vi "FILE New.vi"(0 "New File Path":path, 1 "Prompt":string, 2 "Pattern":string, 3 "Default Name":string, 7 "Append Mode (Overwrite)":T2, 11 "Error In (no error)":errorcluster, 12 "Start Path":path, 13 "Warn on Overwrite (warn)":T1) -> (4 "Refnum":refnum<file>, 8 "File Path":path, 15 "Error Out":errorcluster)   [LabVIEW 2011]
doc: "This vi initializes the creation of a new file, the overwriting of an old file, or the append of new information to an old file depending on the mode enumerations specified.\n\nappend mode: controls the mode that the write operation will take if the file path already exhists. If append is selected then the text (or spreadsheed array) will be appended to the data after the last character in the file. If overwrite is selected then the file will be overwritten by the new data specified.\n\nwarning dialog mode : controls the action of the dialog to warn when a file is about to be overwritten. If 'don't warn' is selected then the file will be automatically overwritten. If the dialog appears and the user chooses not to overwrite then no file operation will take place and no errors will ocurr.\n\nnote: generally canceling out of all dialog boxes will not cause a file error to ocurr, only actual file errors will be flagged."
uses:
  Type Defs/FILE Append Mode Enum.ctl
  Type Defs/FILE Overwrite Warning Enum.ctl
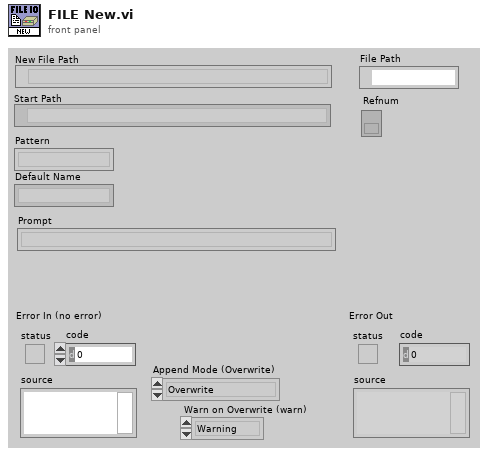
[diagram p1: front panel]
types:
  T1 = typedef "FILE Overwrite Warning Enum.ctl" = enum16{"Warning", "No Warning"}
  T2 = typedef "FILE Append Mode Enum.ctl" = enum16{"Overwrite", "Append"}
  T3 = enum16{"open", "replace", "create", "open or create", "replace or create", "replace or create with confirmation"}
  T4 = enum32{"existing file", "new file", "new or existing file", "existing dir", "new dir", "new or existing dir", "existing file (use LLBs)", "new file (use LLBs)", "new or existing file (use LLBs)", "new or existing file or directory (use LLBs)"}
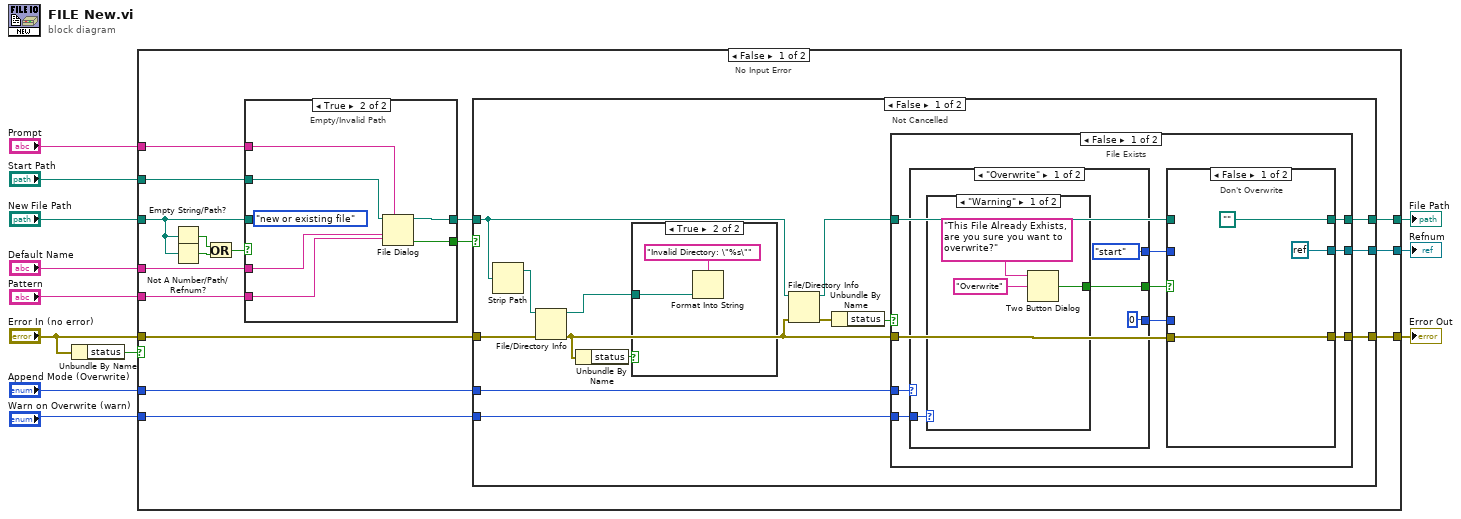
[diagram p0: block diagram]
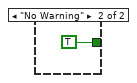
[diagram p3: hidden frame]
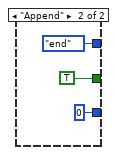
[diagram p4: hidden frame]
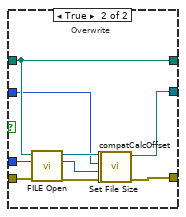
[diagram p5: hidden frame]
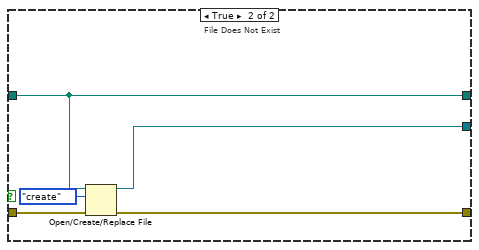
[diagram p6: hidden frame]
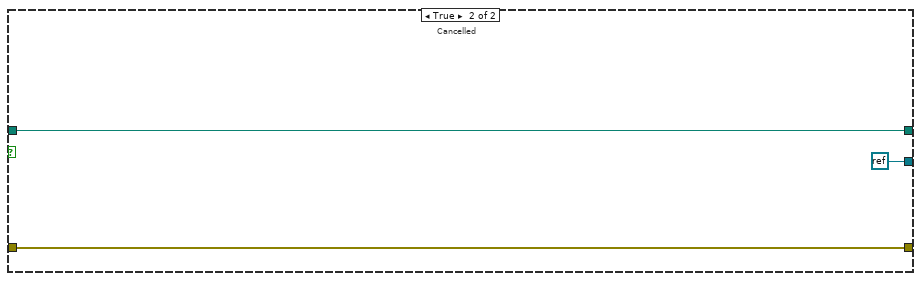
[diagram p7: hidden frame]
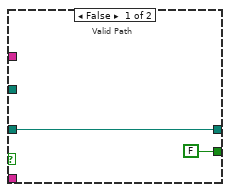
[diagram p8: hidden frame]
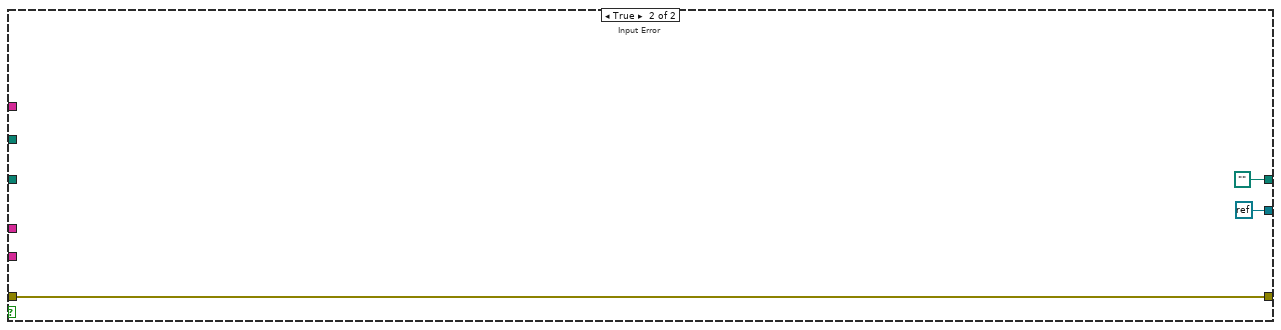
[diagram p9: hidden frame]
diagram:
  n1 = Unbundle By Name("Error In (no error)") -> ("status"=w5:bool)
  n2 = case shown="False" w5 {
    tunnel: [w28 w97] -> w6
    tunnel: "New File Path" -> [w26 _]
    tunnel: "Pattern" -> [w25 _]
    tunnel: "Default Name" -> [w24 _]
    tunnel: "Prompt" -> [w23 _]
    tunnel: "Start Path" -> [w21 _]
    tunnel: "Error In (no error)" -> [w19 w97]
    tunnel: [w16 refnum<k0> refnum] -> w4
    tunnel: [w15 path ""] -> w3
    tunnel: "Append Mode (Overwrite)" -> [w14 _]
    tunnel: "Warn on Overwrite (warn)" -> [w13 _]
    frame False {
      # "No Input Error"
      n3 = Empty String/Path?(string/path=w26) -> (empty?=w17:bool)
      n4 = Not A Number/Path/Refnum?(number/path/refnum=w26) -> (NaN/Path/Refnum?=w18:bool)
      n5 = Or(x=w17, y=w18) -> (x .or. y?=w22:bool)
      n6 = case shown="True" w22 {
        tunnel: w21 -> [_ w95]
        tunnel: [FALSE ("cancelled") w94] -> w20
        tunnel: w23 -> [_ w93]
        tunnel: w24 -> [_ w92]
        tunnel: w25 -> [_ w91]
        tunnel: w26 -> [w89 _]
        tunnel: [w89 w90] -> w27
        frame False {
          # "Valid Path"
        }
        frame True {
          (unwired) T4."new or existing file" ("select mode (2)")
          # "Empty/Invalid Path"
          n7 = File Dialog(6:w91, 7:w93, 9:w92, 11:w95) -> (1:w94:bool, 3:w90:path)  [unwired: 1 in, 4 out]
        }
      }
      n8 = case shown="False" w20 {
        tunnel: w27 -> [w42 w85]
        tunnel: w19 -> [w41 w86]
        tunnel: [w37 refnum<k0> refnum] -> w16
        tunnel: [w36 w86] -> w28
        tunnel: [w35 w85] -> w15
        tunnel: w14 -> [w34 _]
        tunnel: w13 -> [w33 _]
        frame False {
          # "Not Cancelled"
          n9 = Strip Path(path=w42) -> (stripped path=w40:path)  [unwired: 1 out]
          n10 = File/Directory Info(path=w40, error in=w41) -> (path out=w29:path, error out=w31:errorcluster)  [unwired: 5 out]
          n11 = Unbundle By Name(w31) -> ("status"=w30:bool)
          n12 = case shown="True" w30 {
            tunnel: w29 -> [_ w44]
            frame False {
            }
            frame True {
              n13 = Format Into String(format string="Invalid Directory: \"%s\"", w44) -> ()  [unwired: 2 in, 2 out]
            }
          }
          n14 = File/Directory Info(path=w42, error in=w31) -> (path out=w38:path, error out=w32:errorcluster)  [unwired: 5 out]
          n15 = Unbundle By Name(w32) -> ("status"=w39:bool)
          n16 = case shown="False" w39 {
            tunnel: w38 -> [w53 w81]
            tunnel: w31 -> [w54 w84]
            tunnel: [w52 w83] -> w36
            tunnel: [w50 w82] -> w37
            tunnel: [w49 w81] -> w35
            tunnel: w34 -> [w48 _]
            tunnel: w33 -> [w45 _]
            frame False {
              # "File Exists"
              n17 = case shown="\"Overwrite\"" w48 {
                tunnel: [w58 TRUE ("T button?")] -> w51
                tunnel: [enum16{"start", "end", "current"}."start" ("pos mode (0:1)") enum16{"start", "end", "current"}."end" ("pos mode (0:1)")] -> w47
                tunnel: [0 ("pos offset (0)") 0 ("pos offset (0)")] -> w46
                tunnel: w45 -> [w55 _]
                frame "Overwrite" {
                  n18 = case shown="\"Warning\"" w55 {
                    tunnel: [w59 TRUE ("T button?")] -> w58
                    frame "Warning" {
                      n19 = Two Button Dialog(message="This File Already Exhists, are you sure you want to overwrite?", 2:"Overwrite" ("T button name (\"OK\")")) -> (T button?=w59:bool)  [unwired: 1 out]
                    }
                    frame "No Warning" {
                    }
                  }
                }
                frame "Append" {
                }
              }
              n20 = case shown="False" w51 {
                tunnel: w54 -> [w68 w79]
                tunnel: w53 -> [_ w74]
                tunnel: [w68 w76] -> w52
                tunnel: [refnum<k0> refnum w75] -> w50
                tunnel: [path "" w74] -> w49
                tunnel: w47 -> [_ w73]
                tunnel: w46 -> [_ w72]
                frame False {
                  # "Don't Overwrite"
                }
                frame True {
                  # "Overwrite"
                  n21 = call "FILE Open.vi"("Error In (no error)"=w79, "File Path (\" \")"=w74) -> ("Error Out"=w78:errorcluster, "Refnum"=w77:refnum<file>)  [unwired: 3 in, 5 out]
                  n22 = call <vilib>:"compatCalcOffset.vi"("error in"=w78, "pos offset (0)"=w72, "pos mode (0:1)"=w73, "refnum"=w77) -> ("error out"=w71:errorcluster, "offset"=w70:i32, "dup refnum"=w69:refnum<file>)  [unwired: 5 out]
                  n23 = Set File Size(4:w71, 6:w70, 7:w69) -> (0:w76:errorcluster, 3:w75:refnum<file>)
                }
              }
            }
            frame True {
              # "File Does Not Exist"
              n24 = Open/Create/Replace File(file path (use dialog)=w81, error in=w84, operation (0:open)=T3."create") -> (refnum out=w82:refnum<file>, error out=w83:errorcluster)  [unwired: 4 out]
            }
          }
        }
        frame True {
          # "Cancelled"
        }
      }
    }
    frame True {
      # "Input Error"
    }
  }
  "Error Out" <- w6
  "Refnum" <- w4
  "File Path" <- w3
